vi "Split Delimiter.vi"(9 "Delimiter":string=" ", 11 "String In":string) -> (1 "Offset":i32, 3 "After Delimiter":string)   [LabVIEW 2012, in "Intellisense Xcontrol.xctl"]
doc: "Words separated by spaces should be searched for as individual keywords, so this VI reads out the last word from the string, which is everything after the last space."
uses:
  Intellisense Xcontrol.xctl
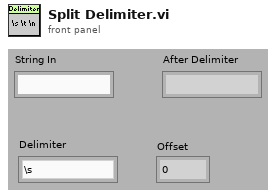
[diagram p1: front panel]
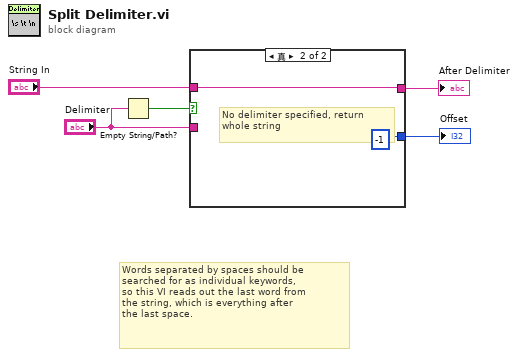
[diagram p0: block diagram]
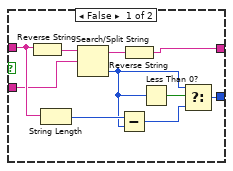
[diagram p2: hidden frame]
diagram:
  # "Words separated by spaces should be\nsearched for as individual keywords,\nso this VI reads out the last word from\nthe string, which is everything after\nthe last space."
  n1 = Empty String/Path?(string/path="Delimiter") -> (empty?=w1:bool)
  n2 = case shown="真" w1 {
    tunnel: [w13 w17] -> w5
    tunnel: "String In" -> [w12 w17]
    tunnel: [w7 -1 ("offset of match")] -> w3
    tunnel: "Delimiter" -> [w6 _]
    frame False {
      n3 = Reverse String(1:w12) -> (0:w15:string)
      n4 = String Length(string=w12) -> (length=w11:i32)
      n5 = Search/Split String(string=w15, search string/char (-)=w6) -> (substring before match=w14:string, offset of match=w9:i32)  [unwired: 1 in, 1 out]
      n6 = Subtract(x=w11, y=w9) -> (x-y=w8:i32)
      n7 = Reverse String(1:w14) -> (0:w13:string)
      n8 = Less Than 0?(x=w9) -> (x < 0?=w10:bool)
      n9 = Select(t=w9, s=w10, f=w8) -> (s? t:f=w7:i32)
    }
    frame True {
      # "No delimiter specified, return\nwhole string"
    }
  }
  "After Delimiter" <- w5
  "Offset" <- w3
